vi "to_json.vi"(8 "error in":errorcluster, 11 "journalJson in":refnum<class "journalJson.lvclass">) -> (0 "error out":errorcluster, 2 "json":string, 3 "journalJson out":refnum<class "journalJson.lvclass">)   [LabVIEW 2020, in "datasources.lvlib" / "journalJson.lvclass"]
uses:
  journalJson.lvclass
  C:/code/labview-client/lv_src/Nominal Client/datasources/datasource/datasource.lvclass
  datasource/datasource.lvclass/datasource.ctl
  journalJson.lvclass/journalJson.ctl
  d89638c6-0f65-4a1b-87d0-923fd0aa4173.vi
  datasource/source.get.vi
  datasource/target.get.vi
  <vilib>/JDP Science/JSONtext/Variant to JSON Text.vi
  <vilib>/JDP Science/JSONtext/support/Format JSON Object.vi
  source/source.lvclass
  target/target.lvclass
  <vilib>/JDP Science/JSONtext/LVClass Serializer/JSONtext LVClass Serializer.lvclass
  <vilib>/JDP Science/JSONtext/JSONtext.lvlib
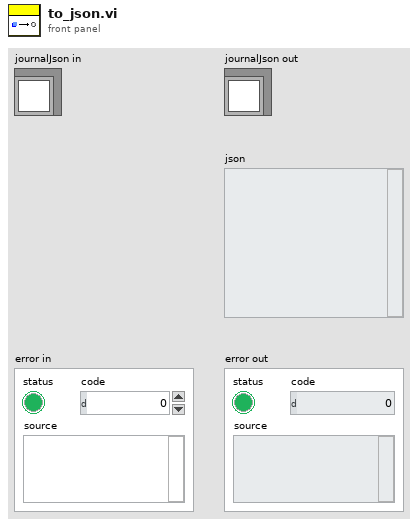
[diagram p1: front panel]
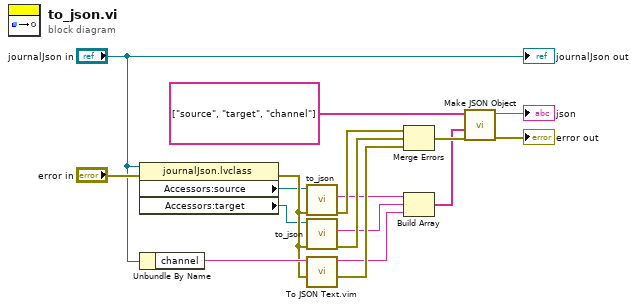
[diagram p0: block diagram]
diagram:
  n1 = property class="journalJson.lvclass"(reference="journalJson in", error in="error in") -> (error out=w8:errorcluster, "Accessors:source"=w3:refnum<class "source.lvclass">, "Accessors:target"=w4:refnum<class "target.lvclass">)  [unwired: 1 out]
  n2 = Unbundle By Name("journalJson in") -> ("channel"=w14:string)
  n3 = call-dynamic "to_json.vi"("error in"=w8, "source in"=w3) -> ("error out"=w17:errorcluster, "json"=w12:string)  [unwired: 7 in, 1 out]
  n4 = call-dynamic "to_json.vi"("error in"=w8, "target in"=w4) -> ("error out"=w16:errorcluster, "json"=w11:string)  [unwired: 7 in, 1 out]
  n5 = call "To JSON Text.vim"("error in (no error)"=w8, "Anything"=w14) -> ("error out"=w15:errorcluster, "<JSON>"=w10:string)  [unwired: 8 in]
  n6 = Merge Errors(w17, w16, w15) -> (w6:errorcluster)
  n7 = Build Array(w12, w11, w10) -> (w1:string[])
  n8 = call <vilib>:"Make JSON Object.vi"("error in (no error)"=w6, "JSON Items"=w1, "Item Names"=string[] ["source", "target", "channel"]) -> ("error out"=→"error out":errorcluster, "<JSON>"=→"json":string)  [unwired: 7 in]
  "journalJson out" <- "journalJson in"
